vi "AutomatedStart.vi"() -> ()   [LabVIEW 2014]
uses:
  <vilib>/userdefined/High Color/nirio_resource_hc.ctl
  TriggerChannel.ctl
  <vilib>/FPGAPlugInAG/PCI-7813R/niLvFpga_Open_PCI-7813R.vi
  <vilib>/rvi/interface/nirviOpenFPGA/nirviOpenFPGA.xnode
  FPGA Bitfiles/W7XBolo2017_FPGATarget_fmain2014_9xlV3GyHFfo.lvbitx
  f_main_2014.vi
  <vilib>/rvi/interface/nirviReadWriteControl/nirviReadWriteControl.xnode
  NiFpgaLv.dll
  <vilib>/Utility/error.llb/Error Cluster From Error Code.vi
  <vilib>/rvi/errors/niLvFpgaAdjustHostInterfaceError.vi
  <vilib>/rvi/interface/nirviMethod/nirviMethod.xnode
  <vilib>/FPGAPlugInAG/PCI-7813R/niLvFpga_Reset_PCI-7813R.vi
panel:
  out "RESET":bool
  out "error out":errorcluster
  out "Operation Watchdog":bool
  out "No. of Software Triggers \ndetected":i16
  out "No. of Hardware Triggers \ndetected":i16
  out "Autmated Start Loop Counter \n(Increasing every 1s)":i32
  out "Timeout ? \n(1s-10s?)":bool
  out "Hardware Trigger \ndetected":bool
  in  "Software Trigger\n(Switch until released)":bool
  in  "Stopp Button":bool
  # "Automated Start W7-X Bolometer DAQ"
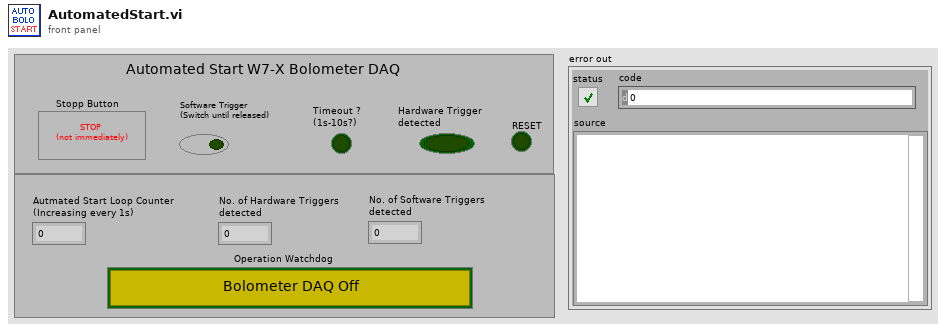
[diagram p1: front panel]
types:
  T1 = typedef "TriggerChannel.ctl" = enum16{"board0 (broken)", "board1 (t = -60sec)", "board2 (t = 0sec)"}
  T2 = enum32{"Invalid", "Standard", "Closed", "Hidden", "Minimized", "Maximized"}
  T3 = typedef "nirio_resource_hc.ctl" = tag
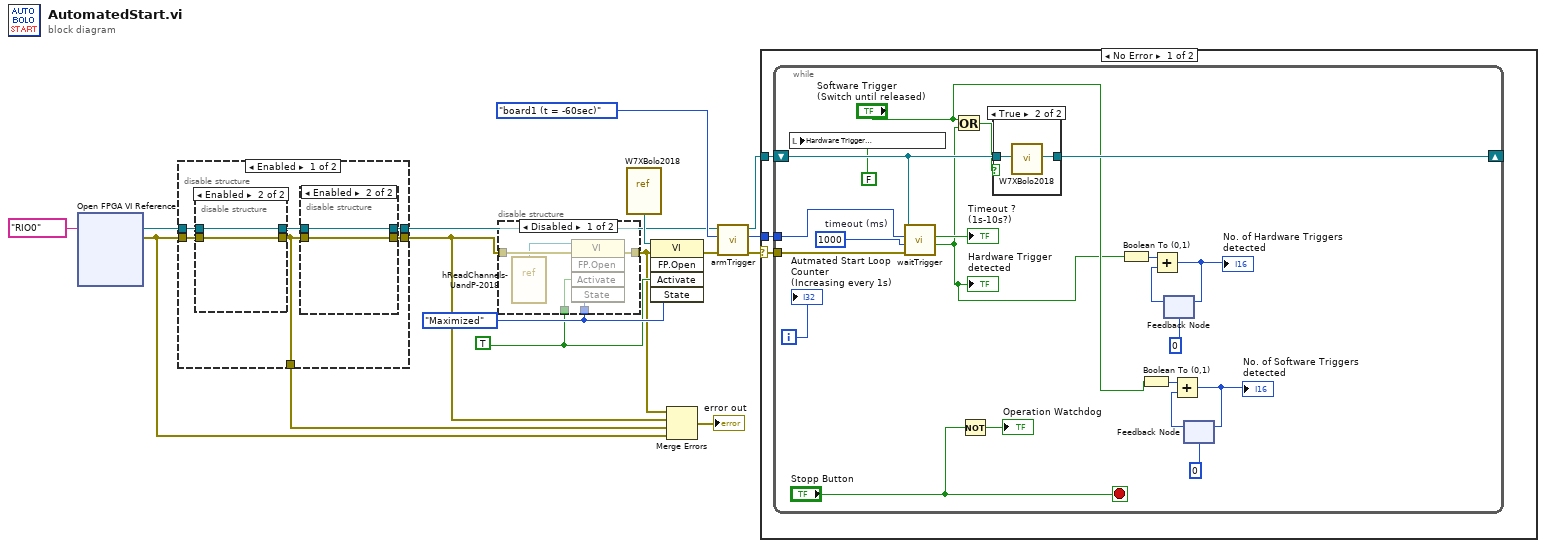
[diagram p0: block diagram]
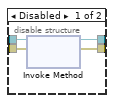
[diagram p2: hidden frame]
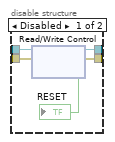
[diagram p3: hidden frame]
diagram:
  w9 = T2."Maximized" ("State")
  w8 = TRUE ("Activate?")
  n1 = xnode "Open FPGA VI Reference"("resource name"=T3 "RIO0") -> ("FPGA VI Reference Out"=w7:refnum<k20>, "error out"=w2:errorcluster)  [unwired: 1 in]
  n2 = disable-structure shown="Enabled" {
    disable-tunnel: w7 -> [w22 w37]
    disable-tunnel: w2 -> [w21 w36]
    disable-tunnel: [w19 w36] -> w4
    disable-tunnel: [w18 w37] -> w6
    disable-tunnel: [w17 _] -> w3
    frame Enabled {
      n3 = disable-structure shown="Enabled" {
        disable-tunnel: w22 -> [w33 w35]
        disable-tunnel: w21 -> [w32 w34]
        disable-tunnel: [w31 w35] -> w20
        disable-tunnel: [w30 w34] -> w17
        frame Disabled {
          n4 = xnode "Read/Write Control"("FPGA VI Reference In"=w33, "error in"=w32) -> ("FPGA VI Reference Out"=w31:refnum<k20>, "error out"=w30:errorcluster, "RESET"=→"RESET":bool)
        }
        frame Enabled {
        }
      }
      n5 = disable-structure shown="Enabled" {
        disable-tunnel: w20 -> [w26 w28]
        disable-tunnel: w17 -> [w25 w27]
        disable-tunnel: [w24 w27] -> w19
        disable-tunnel: [w23 w28] -> w18
        frame Disabled {
          n6 = xnode "Invoke Method"("FPGA VI Reference In"=w26, "error in"=w25) -> ("FPGA VI Reference Out"=w23:refnum<k20>, "error out"=w24:errorcluster)
        }
        frame Enabled {
        }
      }
    }
    frame Disabled {
    }
  }
  n7 = disable-structure shown="Disabled" {
    disable-tunnel: w4 -> [w42 _]
    disable-tunnel: [w41 _] -> w5
    disable-tunnel: w9 -> [w40 _]
    disable-tunnel: w8 -> [w39 _]
    frame Disabled {
      n8 = vi-ref "hReadChannels-UandP-2018.vi"() -> (w38:refnum<vi>)
      n9 = invoke class="VI" method="FP.Open"(reference=w38, error in=w42, "Activate"=w39, "State"=w40) -> (error out=w41:errorcluster)  [unwired: 1 in, 4 out]
    }
    frame Enabled {
    }
  }
  n10 = vi-ref "W7XBolo2018.vi"() -> (w10:refnum<vi>)
  n11 = invoke class="VI" method="FP.Open"(reference=w10, error in=w5, "Activate"=w8, "State"=w9) -> (error out=w15:errorcluster)  [unwired: 1 in, 4 out]
  n12 = Merge Errors(w5, w4, w3, w2) -> (→"error out":errorcluster)
  n13 = call "armTrigger.vi"("error in (no error)"=w15, "Trigger default: board0 (t = 0)"=TriggerChannel."board1 (t = -60sec)", "Refnum in"=w6) -> ("error out"=w14:errorcluster, "IRQ"=w11:i32, "Refnum out"=w12:refnum<k20>)  [unwired: 6 in]
  n14 = case shown="No Error" w14 {
    selector: w14 -> [w43 _]
    tunnel: w12 -> [w45 _]
    tunnel: w11 -> [w44 _]
    frame No Error {
      n15 = while {
        shift-right: [w65] -> _
        shift-left: w45 -> [w66]
        tunnel: w44 -> [w63]
        tunnel: w43 -> [w62]
        i -> [w59]
        stop <- "Stopp Button" stop-if-true
        w64 = 1000  # timeout (ms)
        n16 = local write "Hardware Trigger \ndetected"(FALSE) -> ()
        n17 = call "waitTrigger.vi"("error in (no error)"=w62, "timeout (ms) default: 10s"=w64, "IRQ"=w63, "Refnum in"=w66) -> ("Boolean"=w48:bool, "Timed Out"=→"Timeout ? \n(1s-10s?)":bool)  [unwired: 4 in, 2 out]
        "Hardware Trigger \ndetected" <- w48
        n18 = Or(x="Software Trigger\n(Switch until released)", y=w48) -> (x .or. y?=w54:bool)
        n19 = Not(x="Stopp Button") -> (.not. x?=→"Operation Watchdog":bool)
        n20 = case shown="True" w54 {
          tunnel: w66 -> [w67 w69]
          tunnel: [w67 w68] -> w65
          frame False {
          }
          frame True {
            n21 = call "W7XBolo2018.vi"("FPGA VI Reference In"=w69) -> ("FPGA VI Reference Out"=w68:refnum<k20>)
          }
        }
        n22 = Boolean To (0,1)(Boolean=w48) -> (0, 1=w57:i16)
        n23 = Boolean To (0,1)(Boolean="Software Trigger\n(Switch until released)") -> (0, 1=w52:i16)
        n24 = feedback #1(i16 0) -> (w58:i16)
        n25 = Add(x=w57, y=w58) -> (x+y=w55:i16)
        "No. of Hardware Triggers \ndetected" <- w55
        n26 = feedback-in #1(w55) -> ()
        n27 = feedback #2(i16 0) -> (w53:i16)
        n28 = Add(x=w52, y=w53) -> (x+y=w50:i16)
        "No. of Software Triggers \ndetected" <- w50
        n29 = feedback-in #2(w50) -> ()
        "Autmated Start Loop Counter \n(Increasing every 1s)" <- w59
      }
    }
    frame Error {
    }
  }
